vi "1208LS polling multiple channels AI DI DO.vi"() -> ()   [LabVIEW 2010]
uses:
  <vilib>/ULx/Create Channel.llb/ULx Create Channel (AI-Voltage-Basic).vi
  <vilib>/ULx/Create Channel.llb/ULx Create Channel (DI-Digital Input).vi
  <vilib>/ULx/Create Channel.llb/ULx Create Channel (DO-Digital Output).vi
  <vilib>/ULx/Read.llb/ULx Read (Analog 1D DBL NChan 1Samp).vi
  <vilib>/ULx/Read.llb/ULx Read (Digital U8 1Chan 1Samp).vi
  <vilib>/ULx/Write.llb/ULx Write (Digital U8 1Chan 1Samp).vi
panel:
  out "AI voltage data (from channels 0-3)":dbl[](array[numeric])
  out "Loop Counter":i32
  out "error out":errorcluster
  in  "DO data (byte to port B)":u8 step=1
  out "DI data  (byte from port A)":u8
  in  "stop":bool
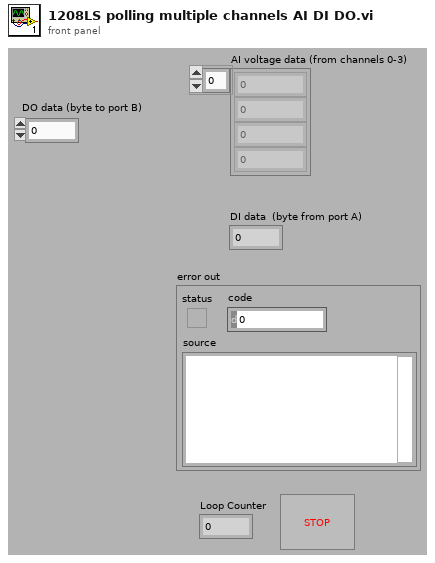
[diagram p1: front panel]
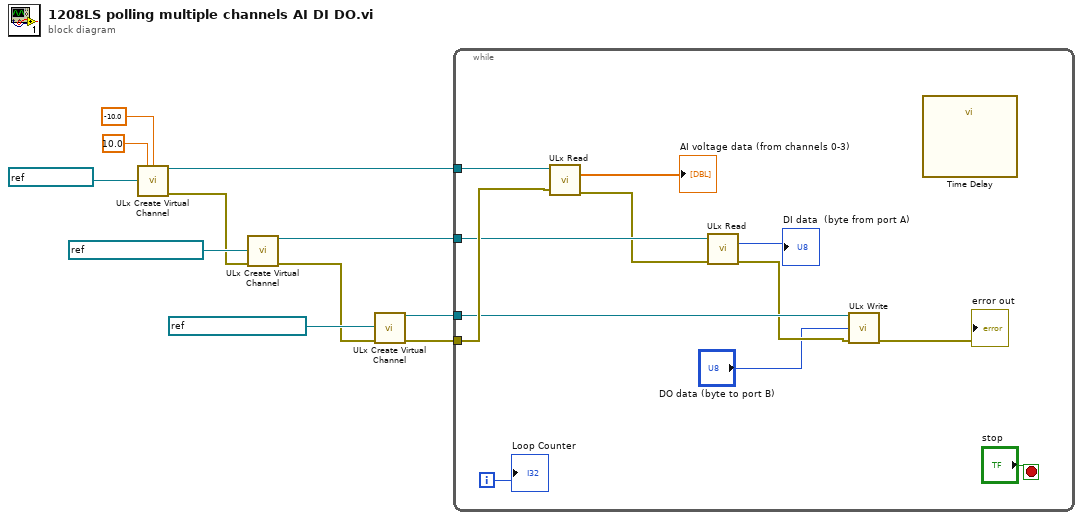
[diagram p0: block diagram]
diagram:
  n1 = call-poly <vilib>:"ULx Create Virtual Channel.vi"("maximum value"=10.0, "minimum value"=-10.0, "physical channels"=refnum<k21> "Dev0/Ai0:3") -> ("task out"=w4:refnum<k24>, "error out"=w8:errorcluster)  [unwired: 11 in]
  n2 = call-poly <vilib>:"ULx Create Virtual Channel.vi"("lines"=refnum<k21> "Dev0/1stPortA/Di0:7", "error in"=w8) -> ("task out"=w2:refnum<k24>, "error out"=w7:errorcluster)  [unwired: 12 in]
  n3 = call-poly <vilib>:"ULx Create Virtual Channel.vi"("lines"=refnum<k21> "Dev0/1stPortB/Do0:7", "error in"=w7) -> ("task out"=w1:refnum<k24>, "error out"=w3:errorcluster)  [unwired: 12 in]
  n4 = while {
    tunnel: w4 -> [w22]
    tunnel: w3 -> [w21]
    tunnel: w2 -> [w20]
    tunnel: w1 -> [w17]
    i -> [w13]
    stop <- "stop" stop-if-true
    n5 = call-poly <vilib>:"ULx Read.vi"("task in"=w22, "error in"=w21) -> ("data"=→"AI voltage data (from channels 0-3)":dbl[], "error out"=w19:errorcluster)  [unwired: 11 in, 1 out]
    n6 = call-poly <vilib>:"ULx Read.vi"("task in"=w20, "error in"=w19) -> ("data"=→"DI data  (byte from port A)":u8, "error out"=w16:errorcluster)  [unwired: 11 in, 1 out]
    n7 = call-poly <vilib>:"ULx Write.vi"("task in"=w17, "data"="DO data (byte to port B)", "error in"=w16) -> ("error out"=→"error out":errorcluster)  [unwired: 10 in, 2 out]
    n8 = call "Time Delay"() -> ()  [unwired: 11 in, 1 out]
    "Loop Counter" <- w13
  }
